vi "Day5-1.vi"() -> ()   [LabVIEW 2021]
panel:
  out "String":string
  out "Map":map{i32, string[]}(c390)
  out "procedure":cluster{i32, i32, i32}[](array[cluster])
  out "initial stacks":map{i32, string[]}(c390)
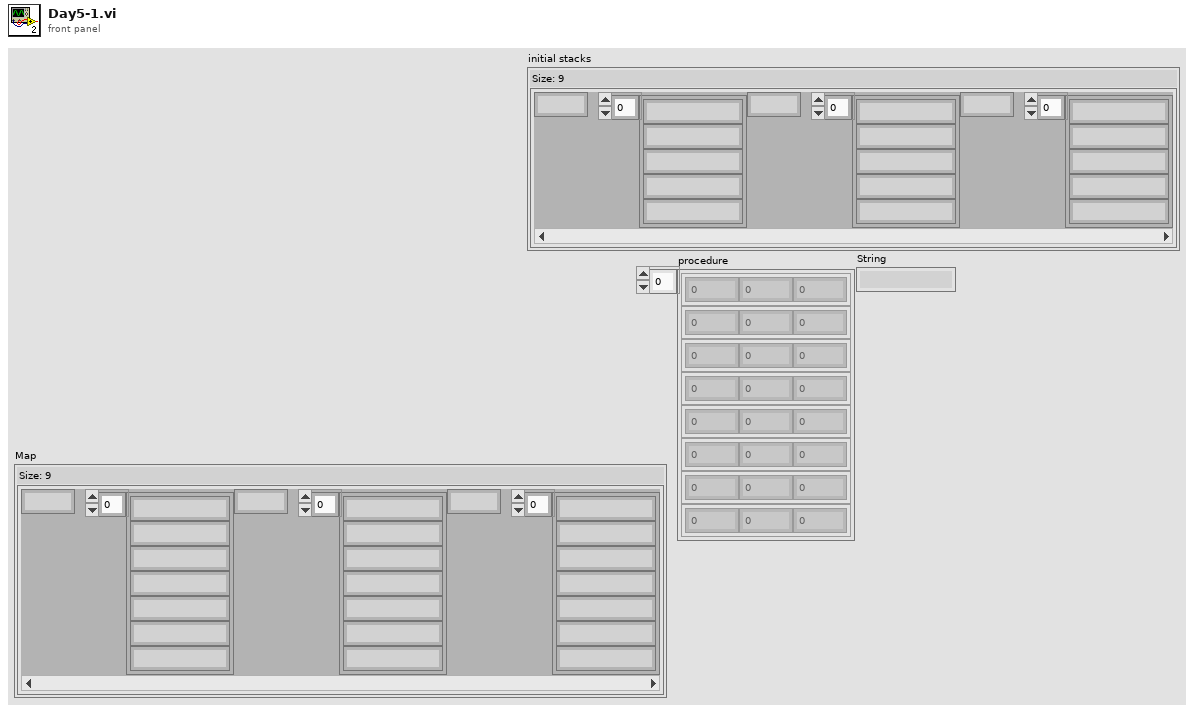
[diagram p1: front panel]
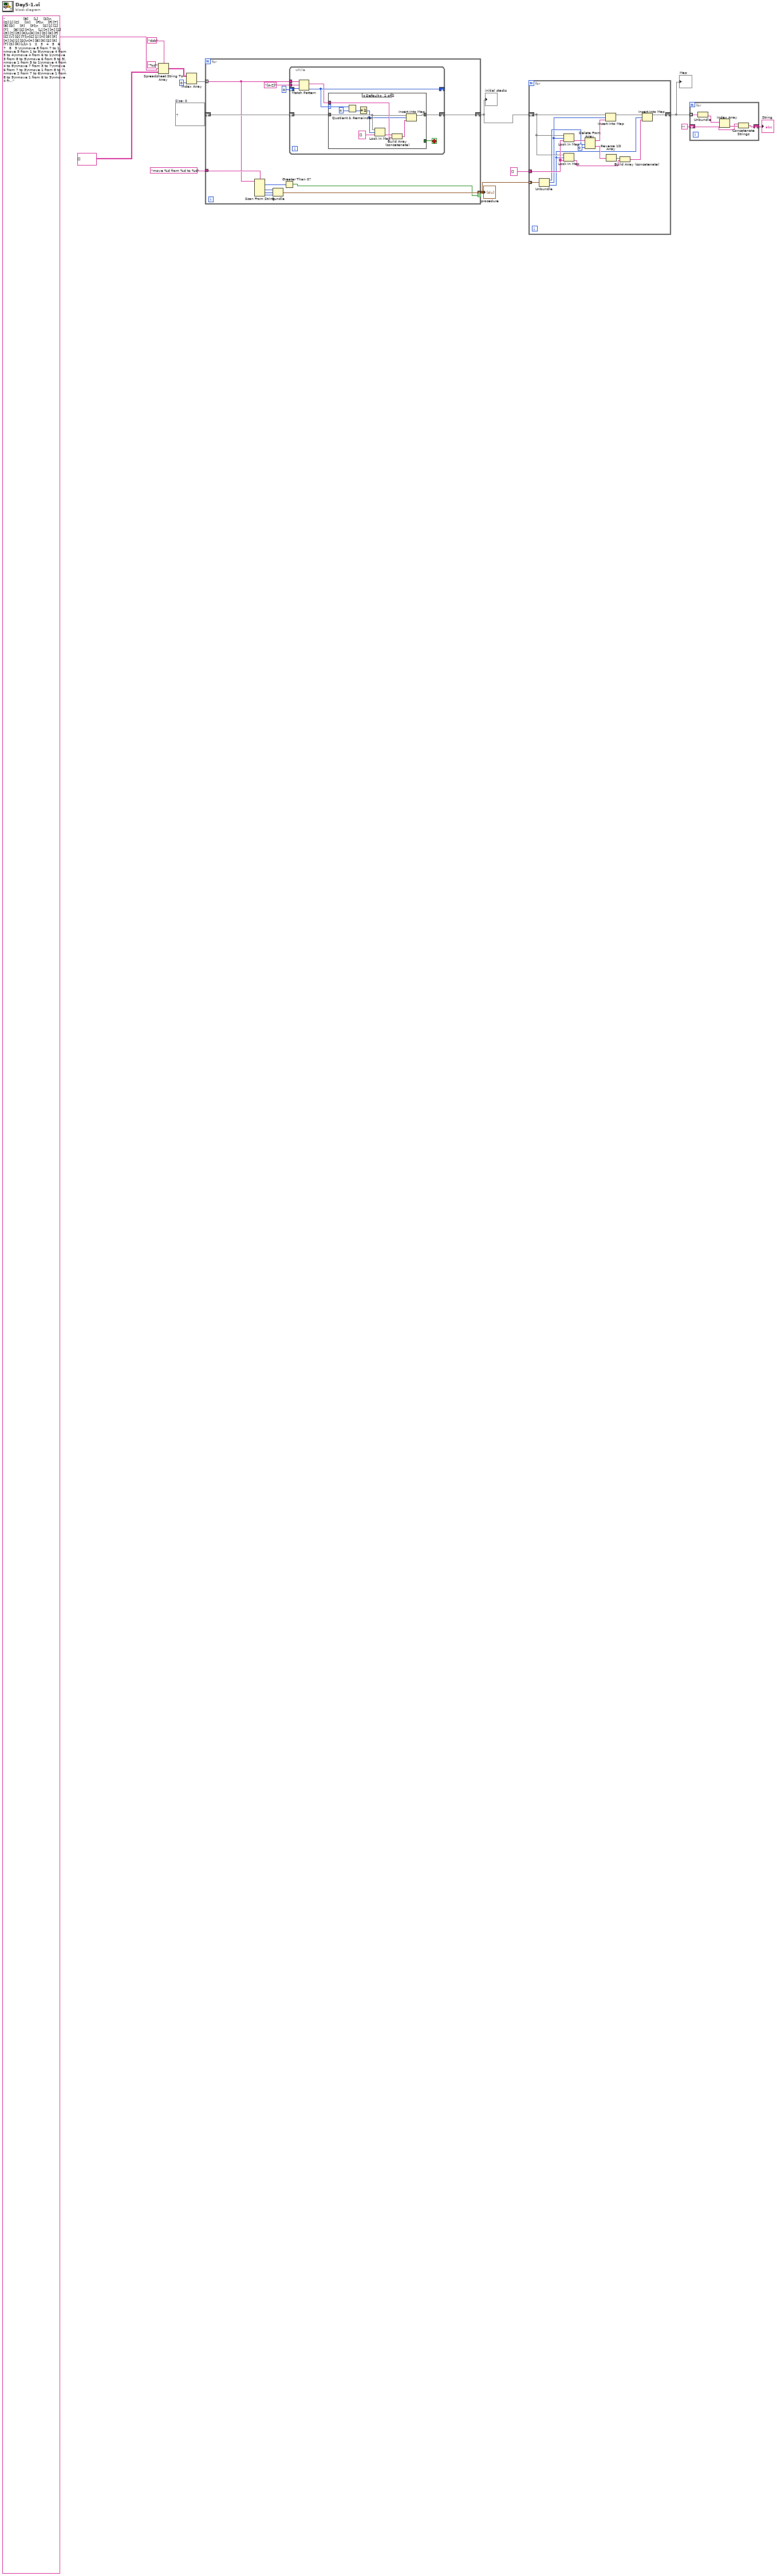
[diagram p0: block diagram]
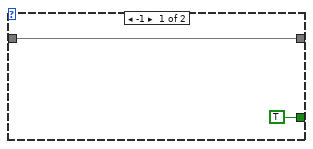
[diagram p2: hidden frame]
diagram:
  w8 = map{i32, string[]} {}  # Size: 0
  n1 = Spreadsheet String To Array(delimiter (Tab)="dsb", format string="%s", spreadsheet string="                [B]     [L]     [S]\n        [Q] [J] [C]     [W]     [F]\n    [F] [T] [B] [D]     [P]     [P]\n    [S] [J] [Z] [T]     [B] [C] [H]\n    [L] [H] [H] [Z] [G] [Z] [G] [R]\n[R] [H] [D] [R] [F] [C] [V] [Q] [T]\n[C] [J] [M] [G] [P] [H] [N] [J] [D]\n[H] [B] [R] [S] [R] [T] [S] [R] [L]\n 1   2   3   4   5   6   7   8   9 \n\nmove 8 from 7 to 1\nmove 9 from 1 to 9\nmove 4 from 5 to 4\nmove 4 from 6 to 1\nmove 3 from 8 to 5\nmove 6 from 5 to 9\nmove 1 from 5 to 1\nmove 4 from 4 to 9\nmove 7 from 3 to 7\nmove 6 from 7 to 3\nmove 1 from 8 to 7\nmove 2 from 7 to 6\nmove 1 from 8 to 9\nmove 1 from 6 to 3\nmove 4 from 3 to 5\nmove 5 from 1 to 3\nmove 1 from 1 to 8\nmove 2 from 3 to 4\nmove 1 from 4 to 1\nmove 7 from 9 to 2\nmove 1 from 6 to 3\nmove 2 from 1 to 9\nmove 20 from 9 to 7\nmove 6 from 4 to 9\nmove 1 from 2 to 9\nmove 6 from 9 to 4\nmove 1 from 4 to 6\nmove 1 from 8 to 6\nmove 1 from 4 to 7\nmove 5 from 2 to 3\nmove 2 from 6 to 4\nmove 3 from 9 to 5\nmove 5 from 3 to 5\nmove 3 from 3 to 8\nmove 3 from 5 to 6\nmove 1 from 9 to 8\nmove 5 from 4 to 5\nmove 3 from 4 to 9\nmove 1 from 8 to 2\nmove 2 from 8 to 2\nmove 11 from 5 to 6\nmove 16 from 7 to 1\nmove 2 from 1 to 7\nmove 14 from 6 to 1\nmove 11 from 1 to 6\nmove 2 from 1 to 4\nmove 4 from 3 to 4\nmove 9 from 2 to 4\nmove 2 from 4 to 8\nmove 2 from 5 to 3\nmove 9 from 4 to 7\nmove 2 from 3 to 2\nmove 1 from 2 to 7\nmove 1 from 8 to 4\nmove 4 from 1 to 4\nmove 1 from 9 to 1\nmove 7 from 4 to 7\nmove 2 from 6 to 5\nmove 1 from 8 to 6\nmove 1 from 4 to 2\nmove 10 from 1 to 6\nmove 5 from 7 to 3\nmove 1 from 4 to 7\nmove 2 from 1 to 2\nmove 2 from 2 to 4\nmove 4 from 3 to 4\nmove 18 from 7 to 6\nmove 6 from 6 to 4\nmove 1 from 7 to 4\nmove 1 from 7 to 6\nmove 11 from 4 to 5\nmove 14 from 5 to 9\nmove 1 from 8 to 7\nmove 8 from 6 to 2\nmove 2 from 4 to 5\nmove 7 from 9 to 1\nmove 6 from 9 to 7\nmove 5 from 1 to 8\nmove 1 from 3 to 6\nmove 10 from 6 to 3\nmove 1 from 9 to 6\nmove 1 from 5 to 4\nmove 4 from 3 to 8\nmove 1 from 5 to 9\nmove 9 from 2 to 3\nmove 1 from 9 to 5\nmove 4 from 8 to 4\nmove 1 from 5 to 3\nmove 5 from 8 to 7\nmove 5 from 7 to 2\nmove 3 from 4 to 1\nmove 8 from 6 to 5\nmove 1 from 7 to 9\nmove 4 from 1 to 3\nmove 2 from 4 to 6\nmove 5 from 5 to 2\nmove 4 from 6 to 9\nmove 1 from 1 to 2\nmove 1 from 5 to 6\nmove 7 from 2 to 8\nmove 5 from 6 to 8\nmove 4 from 7 to 9\nmove 15 from 3 to 9\nmove 1 from 7 to 3\nmove 1 from 5 to 3\nmove 6 from 2 to 6\nmove 1 from 5 to 2\nmove 2 from 3 to 9\nmove 1 from 6 to 8\nmove 5 from 8 to 9\nmove 2 from 3 to 8\nmove 3 from 3 to 6\nmove 11 from 9 to 4\nmove 1 from 2 to 1\nmove 2 from 8 to 4\nmove 1 from 1 to 4\nmove 7 from 4 to 7\nmove 9 from 6 to 3\nmove 4 from 7 to 8\nmove 4 from 7 to 6\nmove 19 from 9 to 4\nmove 7 from 8 to 5\nmove 5 from 3 to 6\nmove 6 from 6 to 9\nmove 3 from 3 to 5\nmove 1 from 3 to 9\nmove 8 from 4 to 5\nmove 2 from 9 to 6\nmove 3 from 8 to 2\nmove 1 from 8 to 4\nmove 1 from 2 to 5\nmove 19 from 4 to 1\nmove 2 from 5 to 7\nmove 2 from 2 to 4\nmove 13 from 5 to 2\nmove 1 from 5 to 1\nmove 2 from 6 to 9\nmove 1 from 8 to 7\nmove 9 from 9 to 3\nmove 2 from 3 to 8\nmove 1 from 4 to 2\nmove 5 from 6 to 7\nmove 1 from 4 to 6\nmove 2 from 8 to 7\nmove 7 from 1 to 5\nmove 1 from 6 to 7\nmove 10 from 1 to 8\nmove 1 from 1 to 3\nmove 1 from 1 to 2\nmove 6 from 5 to 3\nmove 4 from 5 to 3\nmove 5 from 7 to 1\nmove 3 from 1 to 2\nmove 4 from 7 to 5\nmove 8 from 3 to 6\nmove 2 from 1 to 7\nmove 4 from 5 to 8\nmove 7 from 3 to 5\nmove 3 from 7 to 2\nmove 1 from 7 to 3\nmove 12 from 2 to 8\nmove 23 from 8 to 2\nmove 16 from 2 to 6\nmove 1 from 9 to 6\nmove 7 from 5 to 7\nmove 7 from 2 to 4\nmove 2 from 3 to 8\nmove 1 from 1 to 9\nmove 5 from 8 to 1\nmove 2 from 3 to 9\nmove 2 from 7 to 1\nmove 4 from 1 to 3\nmove 4 from 7 to 2\nmove 2 from 1 to 4\nmove 11 from 2 to 9\nmove 3 from 3 to 4\nmove 1 from 9 to 1\nmove 2 from 2 to 7\nmove 4 from 4 to 8\nmove 2 from 9 to 5\nmove 2 from 5 to 7\nmove 4 from 4 to 6\nmove 1 from 3 to 8\nmove 1 from 9 to 8\nmove 4 from 4 to 2\nmove 2 from 1 to 3\nmove 1 from 8 to 4\nmove 2 from 3 to 5\nmove 3 from 9 to 7\nmove 2 from 8 to 9\nmove 1 from 9 to 6\nmove 2 from 7 to 3\nmove 2 from 8 to 1\nmove 1 from 4 to 9\nmove 18 from 6 to 2\nmove 1 from 6 to 5\nmove 1 from 5 to 9\nmove 18 from 2 to 3\nmove 1 from 8 to 7\nmove 2 from 5 to 9\nmove 1 from 1 to 4\nmove 3 from 2 to 1\nmove 9 from 9 to 4\nmove 7 from 4 to 6\nmove 2 from 7 to 3\nmove 2 from 4 to 9\nmove 7 from 6 to 7\nmove 3 from 7 to 2\nmove 7 from 6 to 3\nmove 2 from 6 to 9\nmove 24 from 3 to 9\nmove 2 from 6 to 8\nmove 1 from 4 to 2\nmove 2 from 8 to 5\nmove 31 from 9 to 3\nmove 6 from 7 to 4\nmove 35 from 3 to 7\nmove 1 from 1 to 8\nmove 1 from 5 to 7\nmove 1 from 5 to 4\nmove 1 from 3 to 9\nmove 1 from 8 to 2\nmove 3 from 1 to 7\nmove 7 from 4 to 5\nmove 1 from 9 to 8\nmove 4 from 5 to 6\nmove 2 from 5 to 2\nmove 6 from 2 to 5\nmove 2 from 5 to 7\nmove 2 from 2 to 1\nmove 2 from 5 to 4\nmove 1 from 8 to 4\nmove 3 from 4 to 6\nmove 4 from 6 to 7\nmove 1 from 5 to 2\nmove 2 from 6 to 9\nmove 1 from 6 to 4\nmove 1 from 4 to 8\nmove 2 from 9 to 6\nmove 1 from 8 to 9\nmove 34 from 7 to 9\nmove 6 from 7 to 3\nmove 1 from 7 to 2\nmove 1 from 5 to 8\nmove 1 from 8 to 6\nmove 6 from 7 to 4\nmove 1 from 7 to 3\nmove 7 from 3 to 5\nmove 6 from 4 to 6\nmove 31 from 9 to 1\nmove 3 from 5 to 7\nmove 24 from 1 to 3\nmove 1 from 2 to 4\nmove 3 from 9 to 1\nmove 14 from 3 to 5\nmove 1 from 4 to 3\nmove 1 from 9 to 7\nmove 8 from 3 to 7\nmove 1 from 2 to 9\nmove 7 from 1 to 5\nmove 3 from 6 to 8\nmove 3 from 6 to 1\nmove 1 from 1 to 3\nmove 4 from 3 to 2\nmove 4 from 2 to 3\nmove 2 from 5 to 1\nmove 9 from 7 to 4\nmove 1 from 6 to 5\nmove 1 from 1 to 7\nmove 3 from 8 to 9\nmove 5 from 4 to 2\nmove 3 from 2 to 3\nmove 1 from 2 to 3\nmove 2 from 4 to 1\nmove 2 from 9 to 4\nmove 1 from 9 to 3\nmove 1 from 6 to 1\nmove 1 from 9 to 6\nmove 25 from 5 to 4\nmove 4 from 1 to 9\nmove 2 from 3 to 7\nmove 2 from 6 to 9\nmove 2 from 9 to 5\nmove 6 from 7 to 1\nmove 5 from 3 to 6\nmove 10 from 4 to 3\nmove 10 from 4 to 8\nmove 2 from 4 to 2\nmove 5 from 1 to 9\nmove 2 from 6 to 4\nmove 6 from 9 to 6\nmove 7 from 6 to 4\nmove 3 from 9 to 4\nmove 3 from 2 to 4\nmove 4 from 3 to 8\nmove 2 from 5 to 3\nmove 10 from 4 to 9\nmove 4 from 9 to 7\nmove 5 from 9 to 5\nmove 4 from 5 to 1\nmove 9 from 4 to 6\nmove 10 from 1 to 3\nmove 1 from 5 to 4\nmove 3 from 4 to 5\nmove 2 from 5 to 7\nmove 1 from 7 to 3\nmove 1 from 6 to 9\nmove 11 from 8 to 6\nmove 14 from 6 to 5\nmove 1 from 4 to 7\nmove 7 from 5 to 3\nmove 3 from 5 to 4\nmove 2 from 9 to 5\nmove 2 from 4 to 3\nmove 2 from 7 to 4\nmove 11 from 3 to 9\nmove 2 from 8 to 2\nmove 2 from 2 to 3\nmove 1 from 8 to 2\nmove 1 from 2 to 9\nmove 3 from 4 to 5\nmove 2 from 6 to 9\nmove 1 from 1 to 8\nmove 10 from 9 to 7\nmove 2 from 9 to 3\nmove 23 from 3 to 9\nmove 4 from 6 to 4\nmove 9 from 5 to 6\nmove 1 from 5 to 3\nmove 5 from 6 to 7\nmove 1 from 1 to 7\nmove 1 from 3 to 9\nmove 4 from 6 to 7\nmove 1 from 8 to 7\nmove 1 from 7 to 5\nmove 1 from 5 to 1\nmove 12 from 7 to 6\nmove 9 from 9 to 3\nmove 6 from 6 to 4\nmove 8 from 7 to 3\nmove 3 from 7 to 4\nmove 6 from 3 to 1\nmove 10 from 4 to 8\nmove 10 from 8 to 7\nmove 2 from 3 to 7\nmove 9 from 3 to 8\nmove 2 from 6 to 3\nmove 10 from 7 to 1\nmove 3 from 4 to 6\nmove 5 from 8 to 5\nmove 3 from 5 to 7\nmove 1 from 3 to 2\nmove 1 from 2 to 6\nmove 6 from 9 to 1\nmove 12 from 1 to 3\nmove 3 from 6 to 9\nmove 3 from 1 to 7\nmove 1 from 3 to 2\nmove 7 from 1 to 7\nmove 1 from 2 to 7\nmove 2 from 6 to 4\nmove 1 from 4 to 5\nmove 3 from 8 to 7\nmove 2 from 6 to 3\nmove 2 from 6 to 1\nmove 1 from 3 to 8\nmove 5 from 3 to 4\nmove 2 from 8 to 5\nmove 14 from 7 to 4\nmove 1 from 3 to 2\nmove 1 from 3 to 7\nmove 7 from 7 to 4\nmove 2 from 5 to 3\nmove 2 from 1 to 4\nmove 9 from 4 to 6\nmove 1 from 1 to 2\nmove 4 from 9 to 4\nmove 8 from 9 to 3\nmove 2 from 2 to 7\nmove 13 from 4 to 8\nmove 4 from 4 to 1\nmove 2 from 7 to 6\nmove 12 from 3 to 2\nmove 11 from 2 to 9\nmove 6 from 4 to 9\nmove 18 from 9 to 4\nmove 2 from 1 to 6\nmove 6 from 8 to 1\nmove 13 from 6 to 5\nmove 8 from 4 to 5\nmove 1 from 2 to 9\nmove 8 from 1 to 4\nmove 7 from 4 to 8\nmove 4 from 3 to 5\nmove 10 from 8 to 5\nmove 13 from 5 to 8\nmove 12 from 4 to 5\nmove 2 from 9 to 8\nmove 29 from 5 to 9\nmove 24 from 9 to 2\nmove 23 from 2 to 4\nmove 5 from 9 to 2\nmove 7 from 5 to 7\nmove 1 from 5 to 1\nmove 7 from 4 to 8\nmove 14 from 8 to 1\nmove 5 from 2 to 6\nmove 16 from 4 to 7\nmove 8 from 1 to 6\nmove 1 from 2 to 8\nmove 20 from 7 to 6\nmove 11 from 6 to 4\nmove 3 from 1 to 5\nmove 3 from 4 to 3\nmove 8 from 4 to 9\nmove 8 from 6 to 1\nmove 2 from 1 to 4\nmove 3 from 5 to 2\nmove 12 from 8 to 2\nmove 1 from 7 to 1\nmove 1 from 3 to 5\nmove 1 from 7 to 8\nmove 1 from 7 to 3\nmove 12 from 2 to 8\nmove 13 from 6 to 4\nmove 2 from 1 to 9\nmove 3 from 2 to 6\nmove 3 from 9 to 7\nmove 5 from 9 to 1\nmove 4 from 6 to 4\nmove 2 from 3 to 6\nmove 1 from 5 to 9\nmove 1 from 6 to 7\nmove 9 from 1 to 5\nmove 11 from 8 to 3\nmove 1 from 6 to 8\nmove 3 from 7 to 1\nmove 1 from 8 to 7\nmove 2 from 8 to 9\nmove 7 from 1 to 2\nmove 17 from 4 to 7\nmove 1 from 8 to 6\nmove 4 from 7 to 2\nmove 4 from 9 to 7\nmove 4 from 2 to 3\nmove 1 from 1 to 4\nmove 2 from 4 to 3\nmove 9 from 5 to 4\nmove 1 from 6 to 8\nmove 6 from 2 to 1\nmove 5 from 1 to 9\nmove 9 from 4 to 3\nmove 1 from 4 to 6\nmove 2 from 9 to 7\nmove 1 from 1 to 5\nmove 1 from 2 to 7\nmove 1 from 8 to 9\nmove 1 from 6 to 8\nmove 1 from 5 to 4\nmove 1 from 8 to 7\nmove 23 from 3 to 7\nmove 36 from 7 to 6\nmove 33 from 6 to 1\nmove 1 from 4 to 8\nmove 7 from 1 to 5\nmove 1 from 8 to 1\nmove 3 from 7 to 2\nmove 24 from 1 to 3\nmove 7 from 7 to 3\nmove 3 from 5 to 1\nmove 4 from 5 to 3\nmove 1 from 9 to 8\nmove 2 from 9 to 6\nmove 1 from 8 to 5\nmove 3 from 2 to 5\nmove 30 from 3 to 5\nmove 1 from 6 to 7\nmove 6 from 1 to 8\nmove 7 from 3 to 2\nmove 1 from 7 to 5\nmove 2 from 3 to 2\nmove 2 from 6 to 8\nmove 1 from 6 to 1\nmove 7 from 5 to 8\nmove 8 from 8 to 7\nmove 20 from 5 to 8\nmove 2 from 9 to 7\nmove 8 from 2 to 1\nmove 7 from 7 to 3\nmove 1 from 2 to 1\nmove 3 from 7 to 9\nmove 4 from 8 to 3\nmove 5 from 5 to 6\nmove 1 from 5 to 9\nmove 4 from 9 to 4\nmove 1 from 5 to 9\nmove 2 from 3 to 6\nmove 1 from 5 to 8\nmove 7 from 6 to 3\nmove 1 from 4 to 1\nmove 7 from 3 to 2\nmove 3 from 3 to 5\nmove 2 from 4 to 7", array type (2D Dbl)=string[][] []) -> (array=w11:string[][])
  n2 = Index Array(array=w11, index (col)=0 ("disabled index (col)")) -> (element=w9:string[])  [unwired: 1 in]
  n3 = for {
    tunnel: w9 -> [w22] mode=indexing
    shift-right: [w24] -> w6
    shift-left: w8 -> [w25]
    tunnel: "move %d from %d to %d" ("format string") -> [w23]
    tunnel: [w17] -> w5 mode=indexing if=w16
    n4 = Scan From String(format string=w23, input string=w22) -> (offset past scan=w21:u32, output 1=w20:i32, output 2=w19:i32, output 3=w18:i32)  [unwired: 5 in, 2 out]
    n5 = Bundle(w20, w19, w18) -> (w17:cluster{i32, i32, i32})  [unwired: 1 in]
    n6 = Greater Than 0?(x=w21) -> (x > 0?=w16:bool)
    n7 = while {
      tunnel: w22 -> [w35]
      tunnel: "[A-Z]" ("regular expression") -> [w34]
      shift-right: [w32] -> _
      shift-left: 0 ("offset past match") -> [w33]
      shift-right: [w29] -> w24
      shift-left: w25 -> [w30]
      stop <- w28 stop-if-true
      n8 = Match Pattern(string=w35, regular expression=w34, offset (0)=w33) -> (match substring=w31:string, offset past match=w32:i32)  [unwired: 2 out]
      n9 = case shown="Default" w32 {
        selector: w32 -> [_ w47]
        tunnel: w31 -> [_ w41]
        tunnel: w30 -> [w37 w42]
        tunnel: [w37 w38] -> w29
        tunnel: [TRUE _] -> w28
        frame -1 {
        }
        frame Default {
          n10 = Quotient & Remainder(x=w47, y=4) -> (floor(x/y)=w45:i32)  [unwired: 1 out]
          n11 = Increment(x=w45) -> (x+1=w39:i32)
          n12 = Look In Map(map=w42, key=w39, default value=string[] []) -> (value=w43:string[])  [unwired: 1 out]
          n13 = Build Array (concatenate)(w43, w41) -> (w40:string[])
          n14 = Insert Into Map(map in=w42, key=w39, value=w40) -> (map out=w38:map{i32, string[]})  [unwired: 2 out]
        }
      }
    }
  }
  "initial stacks" <- w6
  "procedure" <- w5
  n15 = for {
    shift-right: [w49] -> w3
    shift-left: w6 -> [w58]
    tunnel: w5 -> [w61] mode=indexing
    tunnel: string[] [] ("default value") -> [w62]
    n16 = Unbundle(w61) -> (w59:i32, w57:i32, w50:i32)
    n17 = Look In Map(map=w58, key=w57, default value=w62) -> (value=w60:string[])  [unwired: 1 out]
    n18 = Look In Map(map=w58, key=w50, default value=w62) -> (value=w52:string[])  [unwired: 1 out]
    n19 = Delete From Array(array=w60, length=w59, index=0) -> (deleted portion=w54:string[], array with subset deleted=w56:string[])
    n20 = Insert Into Map(map in=w58, key=w57, value=w56) -> (map out=w55:map{i32, string[]})  [unwired: 2 out]
    n21 = Reverse 1D Array(array=w54) -> (reversed array=w53:string[])
    n22 = Build Array (concatenate)(w53, w52) -> (w51:string[])
    n23 = Insert Into Map(map in=w55, key=w50, value=w51) -> (map out=w49:map{i32, string[]})  [unwired: 2 out]
  }
  "Map" <- w3
  n24 = for {
    tunnel: w3 -> [w67] mode=indexing
    shift-right: [w63] -> w1
    shift-left: "" -> [w64]
    n25 = Unbundle(w67) -> (w66:string[])  [unwired: 1 out]
    n26 = Index Array(array=w66) -> (element=w65:string)  [unwired: 1 in]
    n27 = Concatenate Strings(w64, w65) -> (w63:string)
  }
  "String" <- w1
